vi "generate_waveform.vi"(8 "Ramp parameters XY":T1, 9 "Cycle parameters XY":T9={"Cycle parameters X"={"Imaging cycles"=285714, "Settling cycles"=71429, "Resting cycles"=42857, "Phase advance per cycle"=0.0001399517059326172, "Initial Phase"=0.00286865234375}, "Cycle parameters Y"={"Imaging cycles"=285714, "Settling cycles"=71429, "Resting cycles"=42857, "Phase advance per cycle"=0.0001399517059326172, "Initial Phase"=0.00286865234375}}, 10 "Cycle counters XY In":T7, 11 "Scan counters in":T6 {"Current part of waveform" items=["Imaging", "Settling", "Resting"]}) -> (0 "In range":bool, 1 "Waveform out":cluster{"Coerced Out":u16, "Coerced Out":u16}, 2 "Cycle counters XY out":T7, 3 "Scan counters out":T6 {"Current part of waveform" items=["Imaging", "Settling", "Resting"]})   [LabVIEW 2011]
uses:
  typedefs/cycle_parameters_XY_cluster.ctl
  typedefs/cycle_parameters_cluster.ctl
  typedefs/cycle_counters_XY_cluster.ctl
  typedefs/cycle_counters_cluster.ctl
  typedefs/scan_counters_cluster.ctl
  typedefs/ramp_parameters_XY_cluster.ctl
  typedefs/ramp_parameters_cluster.ctl
  typedefs/ramp_type_enum.ctl
  typedefs/linear_ramp_parameters_cluster.ctl
  typedefs/sine_ramp_parameters_cluster.ctl
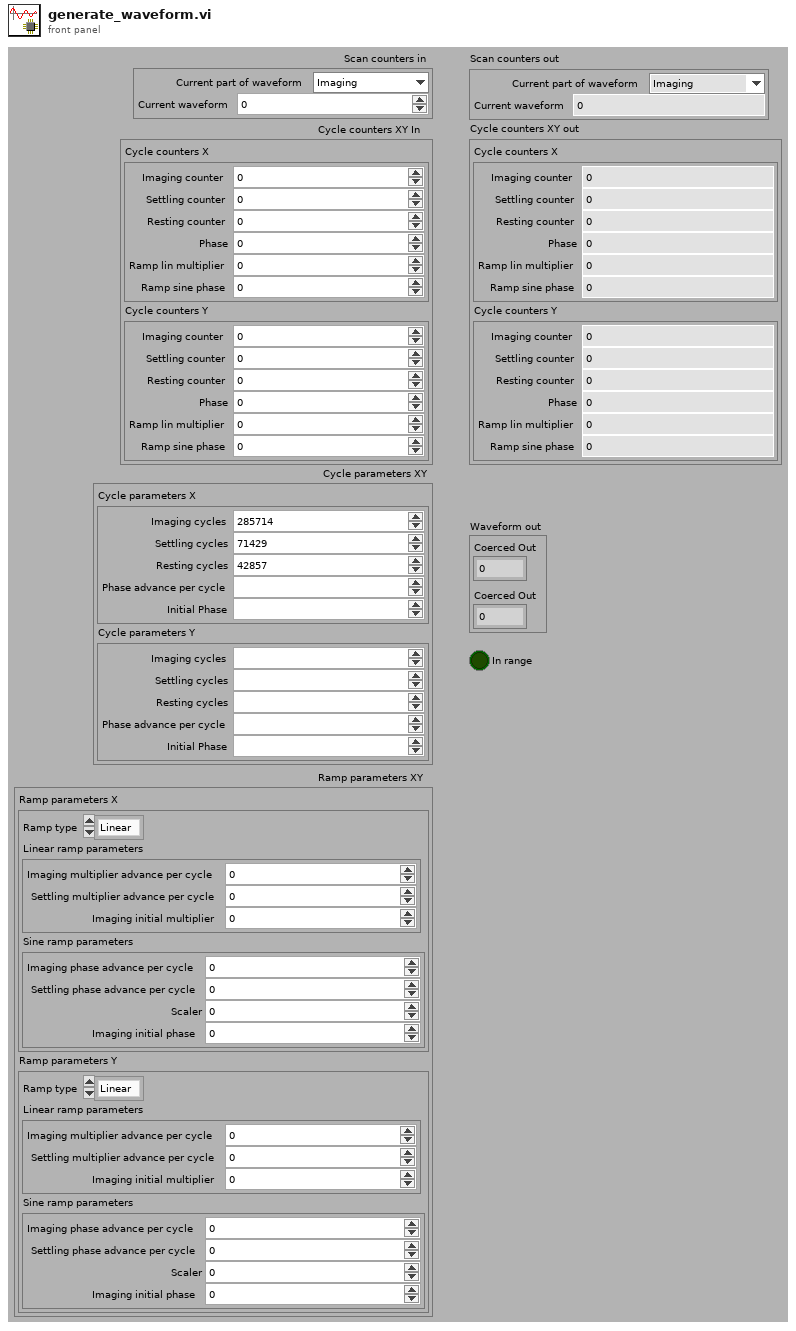
[diagram p1: front panel]
types:
  T1 = typedef "ramp_parameters_XY_cluster.ctl" = cluster{"Ramp parameters X":T2, "Ramp parameters Y":T2}
  T2 = typedef "ramp_parameters_cluster.ctl" = cluster{"Ramp type":T3, "Linear ramp parameters":T4, "Sine ramp parameters":T5}
  T3 = typedef "ramp_type_enum.ctl" = enum8{"Linear", "Sine"}
  T4 = typedef "linear_ramp_parameters_cluster.ctl" = cluster{"Imaging multiplier advance per cycle":fxp<+/-,32,0>, "Settling multiplier advance per cycle":fxp<+/-,32,0>, "Imaging initial multiplier":fxp<+/-,43,12>}
  T5 = typedef "sine_ramp_parameters_cluster.ctl" = cluster{"Imaging phase advance per cycle":fxp<+,32,0>, "Settling phase advance per cycle":fxp<+,32,0>, "Scaler":fxp<+,43,12>, "Imaging initial phase":fxp<+,32,1>}
  T6 = typedef "scan_counters_cluster.ctl" = cluster{"Current part of waveform":u8, "Current waveform":u16}
  T7 = typedef "cycle_counters_XY_cluster.ctl" = cluster{"Cycle counters X":T8, "Cycle counters Y":T8}
  T8 = typedef "cycle_counters_cluster.ctl" = cluster{"Imaging counter":i32, "Settling counter":i32, "Resting counter":i32, "Phase":fxp<+,32,1>, "Ramp lin multiplier":fxp<+/-,43,12>, "Ramp sine phase":fxp<+,32,1>}
  T9 = typedef "cycle_parameters_XY_cluster.ctl" = cluster{"Cycle parameters X":T10, "Cycle parameters Y":T10}
  T10 = typedef "cycle_parameters_cluster.ctl" = cluster{"Imaging cycles":i32, "Settling cycles":i32, "Resting cycles":i32, "Phase advance per cycle":fxp<+,32,0>, "Initial Phase":fxp<+,32,1>}
  T11 = typedef "current_ramp_values_cluster.ctl" = cluster{"Lin multiplier advance per cycle":fxp<+/-,32,0>, "Sine phase advance per cycle":fxp<+,32,0>, "Sine scaler":fxp<+,43,12>}
  T12 = cluster{"Coerced U16 Out":u16, "Coerced U16 Out":u16}
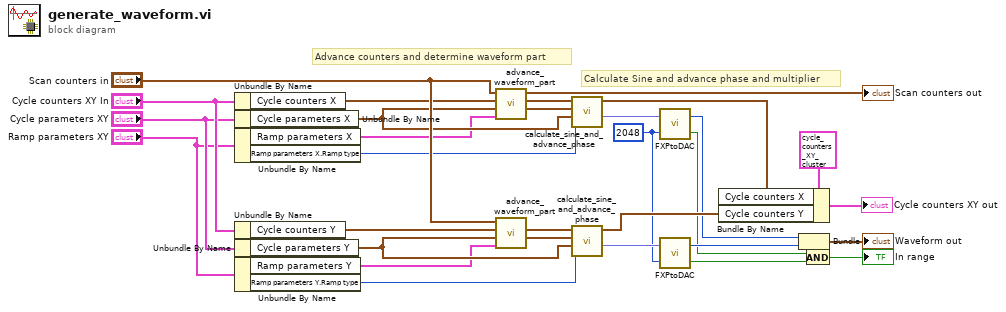
[diagram p0: block diagram]
diagram:
  w1 = i16 2048 ("Offset")
  # "Calculate Sine and advance phase and multiplier"
  # "Advance counters and determine waveform part"
  n1 = Unbundle By Name("Cycle counters XY In") -> ("Cycle counters X"=w23:T8)
  n2 = Unbundle By Name("Cycle parameters XY") -> ("Cycle parameters X"=w10:T10)
  n3 = Unbundle By Name("Ramp parameters XY") -> ("Ramp parameters X"=w6:T2, "Ramp parameters X.Ramp type"=w3:T3)
  n4 = Unbundle By Name("Cycle counters XY In") -> ("Cycle counters Y"=w22:T8)
  n5 = Unbundle By Name("Cycle parameters XY") -> ("Cycle parameters Y"=w7:T10)
  n6 = Unbundle By Name("Ramp parameters XY") -> ("Ramp parameters Y"=w4:T2, "Ramp parameters Y.Ramp type"=w2:T3)
  n7 = call "advance_waveform_part.vi"("Ramp parameters"=w6, "Cycle parameters"=w10, "Cycle counters in"=w23, "Scan counters in"="Scan counters in") -> ("Current ramp values"=w9:T11, "Cycle counters out"=w20:T8, "Scan counters out"=→"Scan counters out":T6)  [unwired: 5 in]
  n8 = call "advance_waveform_part.vi"("Ramp parameters"=w4, "Cycle parameters"=w7, "Cycle counters in"=w22, "Scan counters in"="Scan counters in") -> ("Current ramp values"=w8:T11, "Cycle counters out"=w19:T8)  [unwired: 5 in, 1 out]
  n9 = call "calculate_sine_and_advance_phase.vi"("Ramp type"=w3, "Cycle parameters in"=w10, "Current ramp values"=w9, "Cycle counters in"=w20) -> ("Ramped sine"=w18:fxp<+/-,16,12>, "Cycle counters out"=w25:T8)  [unwired: 6 in]
  n10 = call "calculate_sine_and_advance_phase.vi"("Ramp type"=w2, "Cycle parameters in"=w7, "Current ramp values"=w8, "Cycle counters in"=w19) -> ("Ramped sine"=w17:fxp<+/-,16,12>, "Cycle counters out"=w24:T8)  [unwired: 6 in]
  n11 = call "FXPtoDAC.vi"("Offset"=w1, "FXP In"=w18) -> ("In Range?"=w13:bool, "Coerced U16 Out"=w16:u16)
  n12 = call "FXPtoDAC.vi"("Offset"=w1, "FXP In"=w17) -> ("In Range?"=w12:bool, "Coerced U16 Out"=w15:u16)
  n13 = Bundle By Name(cluster=T7 {"Cycle counters X"={"Imaging counter"=0, "Settling counter"=0, "Resting counter"=0, "Phase"=0.0, "Ramp lin multiplier"=0.0, "Ramp sine phase"=0.0}, "Cycle counters Y"={"Imaging counter"=0, "Settling counter"=0, "Resting counter"=0, "Phase"=0.0, "Ramp lin multiplier"=0.0, "Ramp sine phase"=0.0}} ("FPGA Waveform Counters Out"), "Cycle counters X"=w25, "Cycle counters Y"=w24) -> (→"Cycle counters XY out":T7)
  n14 = Bundle("Coerced U16 Out"=w16, "Coerced U16 Out"=w15) -> (→"Waveform out":T12)  [unwired: 1 in]
  n15 = And(x=w13, y=w12) -> (x .and. y?=→"In range":bool)
